vi "Performance Test.vi"() -> ()   [LabVIEW 2021]
uses:
  ChannelCommon/typedef/Benchmark Stats.ctl
  ChannelCommon/typedef/Datatype Waveform.ctl
  CIFChannels/Typedef/Direction.ctl
  ChannelCommon/typedef/FIFO Config.ctl
  CIF_NIChn_FIFO_DAQ_DVR.lvclass
  D:/dev/Packages/Channel_Manager/src/CIFChannels/CIFChannels.lvclass
  <vilib>/Platform/TimedLoop/XDataNode/timing_clust.ctl
  <vilib>/Platform/TimedLoop/XDataNode/nitl_modes.ctl
  <vilib>/Platform/TimedLoop/XDataNode/wakeup.ctl
  ChannelCommon/typedef/TimeStamps.ctl
  CIFChannels/CIFChannels.lvclass/CIFChannels.ctl
  <vilib>/CIF Foundation/CIF Utilities/Statistics/I64/Stats_I64_CIF_U.lvclass/Stats_I64_CIF_U.ctl
  <vilib>/CIF Foundation/CIF Utilities/DataTypes/Flatten U64.vi
  <vilib>/CIF Foundation/CIF Utilities/Statistics/I64/Get Stats.vi
  <vilib>/Platform/TimedLoop/XDataNode/XDataNode.xnode
  <vilib>/Platform/TimedLoop/XDataNode/XDNodeRunTimeDep.lvlib
  CIFChannels/CIFChannels.lvclass
  ChannelCommon/ChannelCommon.lvlib
panel:
  out "Timeout RW Inline":bool
  out "Write (us) 3":T1
  out "Flatten (us) 3":T1
  out "Data Out":T2[](array[typedef])=[{"measurement"=array[200001 elements], "dT"=43.0, "Timestamp"=2, "Read Lock"=FALSE}, {"measurement"=array[200001 elements], "dT"=34.0, "Timestamp"=1, "Read Lock"=FALSE}]
  out "Read (us) 3":T1
  out "Unflatten (us) 3":T1
  out "Flatten (us) TO":T1
  out "Channel R/W (us) TO":T1
  out "Flatten (us)":T1
  out "Channel R/W (us)":T1
  out "avg TO":dbl
  out "max TO":dbl
  out "timed out? 3":bool
  out "timed out?":bool
  out "avg channel":dbl
  out "max channel":dbl
  out "pass":bool
  out "error out":errorcluster
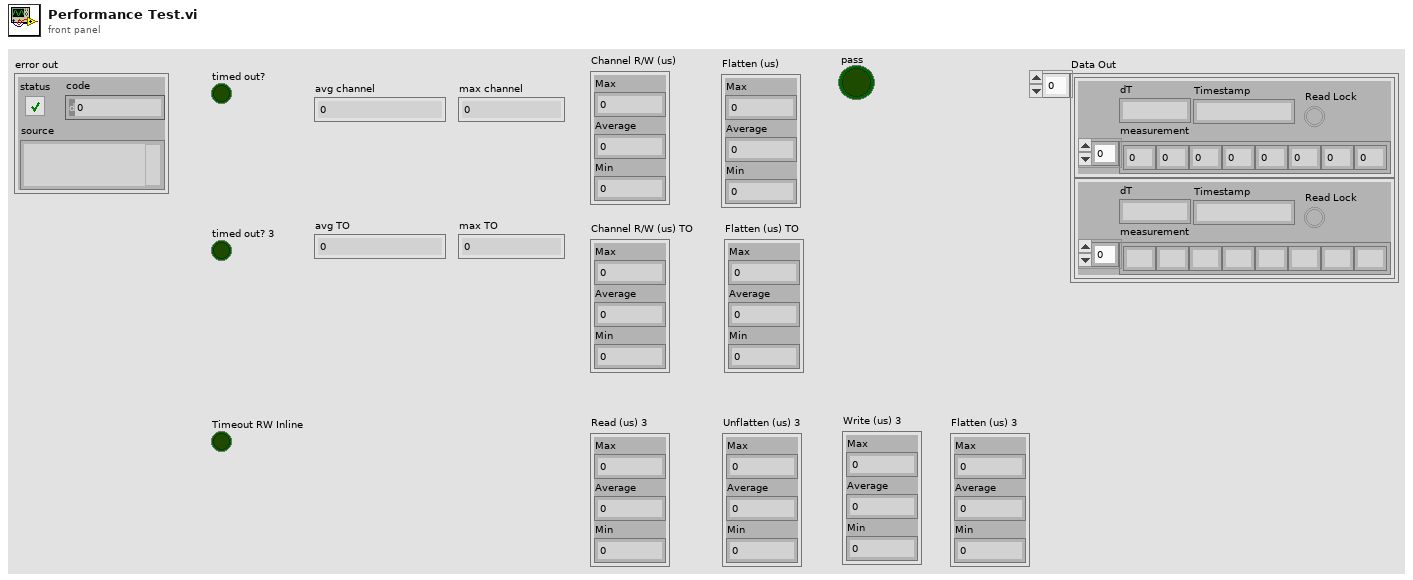
[diagram p1: front panel]
types:
  T1 = typedef "ChannelCommon.lvlib/Benchmark Stats.ctl" = cluster{"Max":i64, "Average":dbl, "Min":i64}
  T2 = typedef "ChannelCommon.lvlib/Datatype Waveform.ctl" = cluster{"measurement":dbl[], "dT":dbl, "Timestamp":i64, "Read Lock":bool}
  T3 = typedef "ChannelCommon.lvlib/FIFO Config.ctl" = cluster{"Max Bytes/Msg":u64, "Max Msg/FIFO":u64, "Flags":u64}
  T4 = typedef "CIFChannels.lvclass/Direction.ctl" = enum16{"Publisher", "Subscriber"}
  T5 = typedef "ChannelCommon.lvlib/TimeStamps.ctl" = cluster{"ClockID":u8, "T0":i64, "T_Out":i64}
  T6 = typedef "XDNodeRunTimeDep.lvlib/timing_clust.ctl" = cluster{"Expected End [f-1]":u64, "Actual End [f-1]":u64, "Finished Late? [f-1]":bool, "Expected End [i-1]":u64, "Actual End [i-1]":u64, "Finished Late? [i-1]":bool, "Expected Start [i]":u64, "Actual Start [i]":u64, "Expected Start [f]":u64, "Actual Start [f]":u64, "Source Name":string, "Structure Name":string, "Period":i64, "Deadline":i64, "Offset":i64, "Start":i64, "Priority":i32, "Timeout":i32, "Mode":T7, "Wakeup Reason":T8, "Error":errorcluster, "Source Type":string, "Secondary Source Type":string, "Global End Time":u64, "Global Start Time":u64, "Frame Duration":u64, "Iteration Duration":u64, "Assigned CPU":i32, "I/O Scan Engine Mode":u32}
  T7 = typedef "XDNodeRunTimeDep.lvlib/nitl_modes.ctl" = enum32{"No Change", "Process missed periods, maintain original phase", "Discard missed periods, maintain original phase", "Process missed periods, ignore original phase", "Discard missed periods, ignore original phase"}
  T8 = typedef "XDNodeRunTimeDep.lvlib/wakeup.ctl" = enum32{"Normal", "Aborted", "Asynchronous wakeup", "Timing source error", "Timed loop error", "Timeout"}
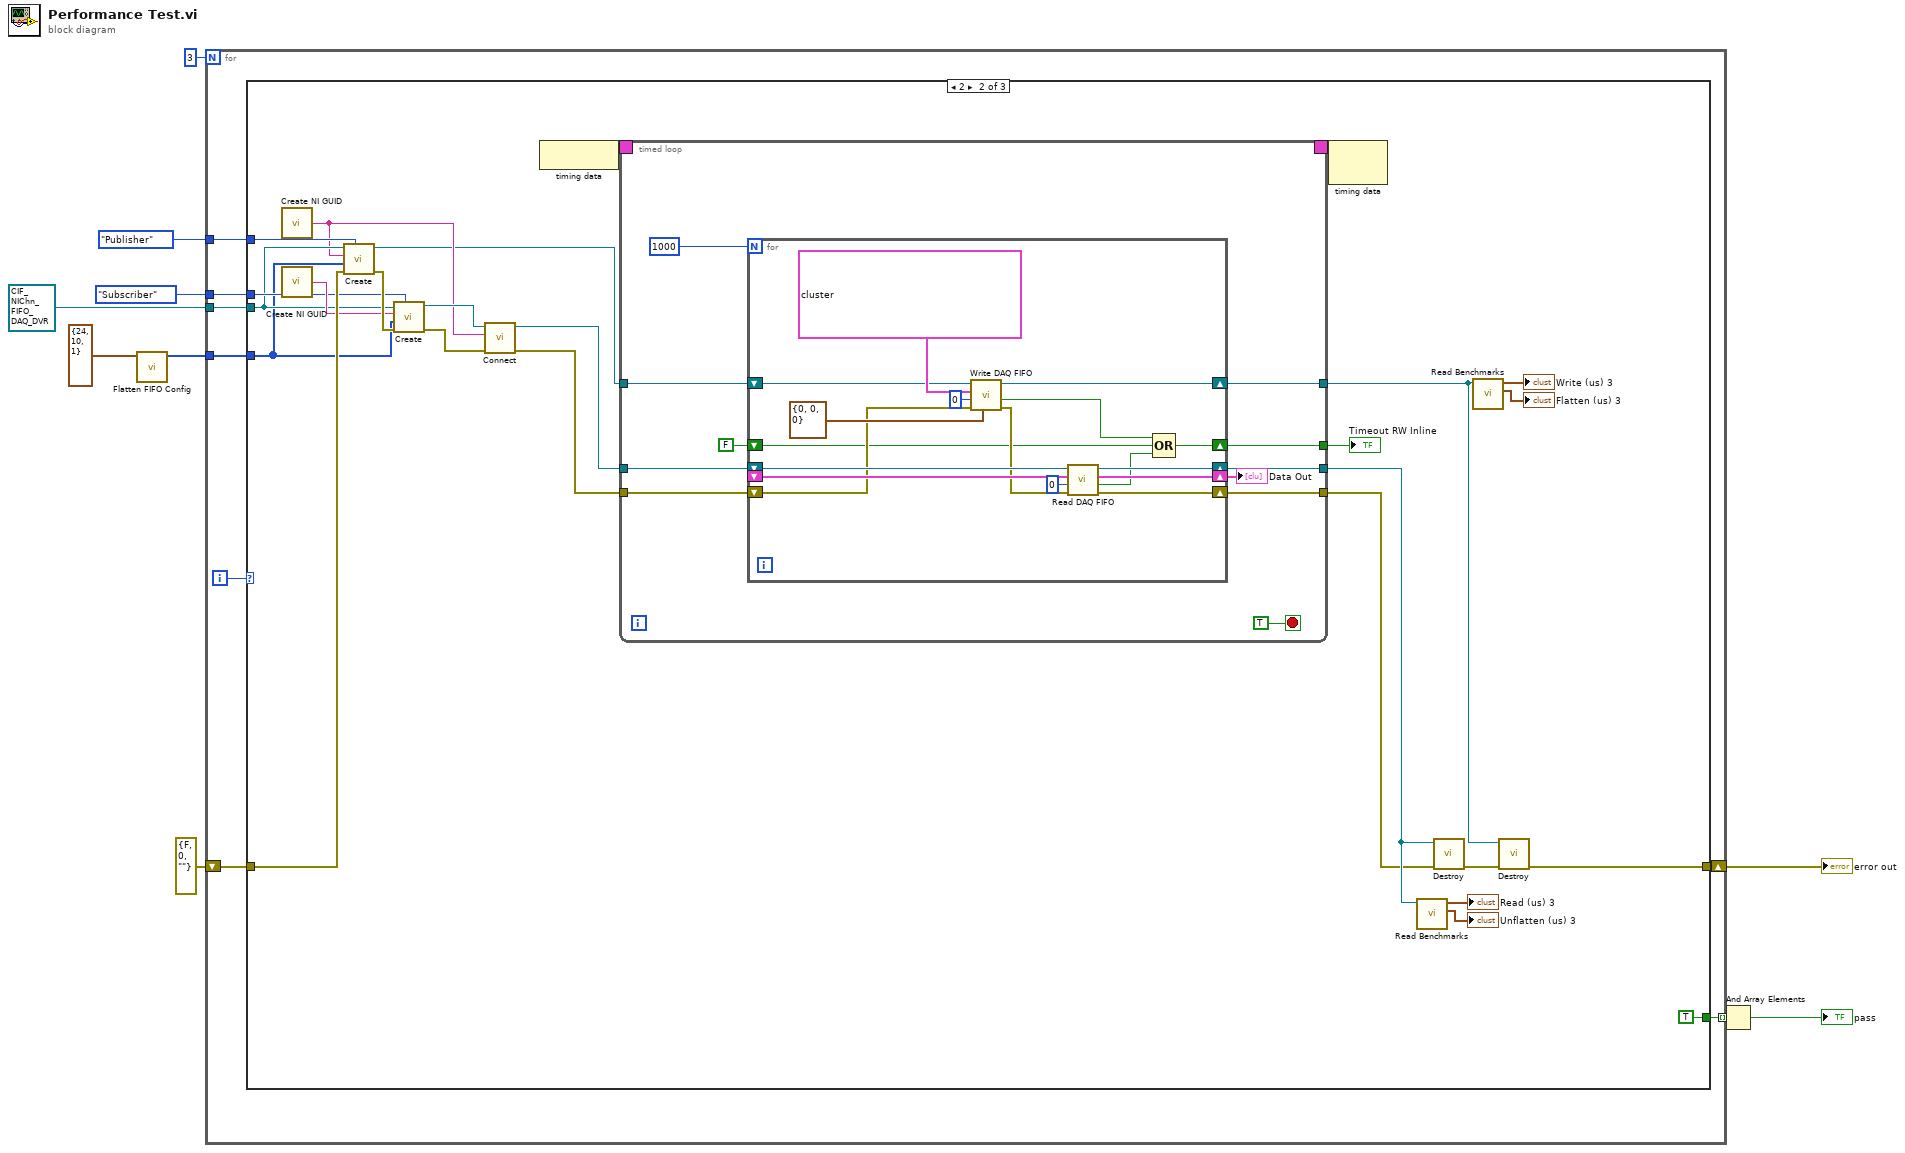
[diagram p0: block diagram]
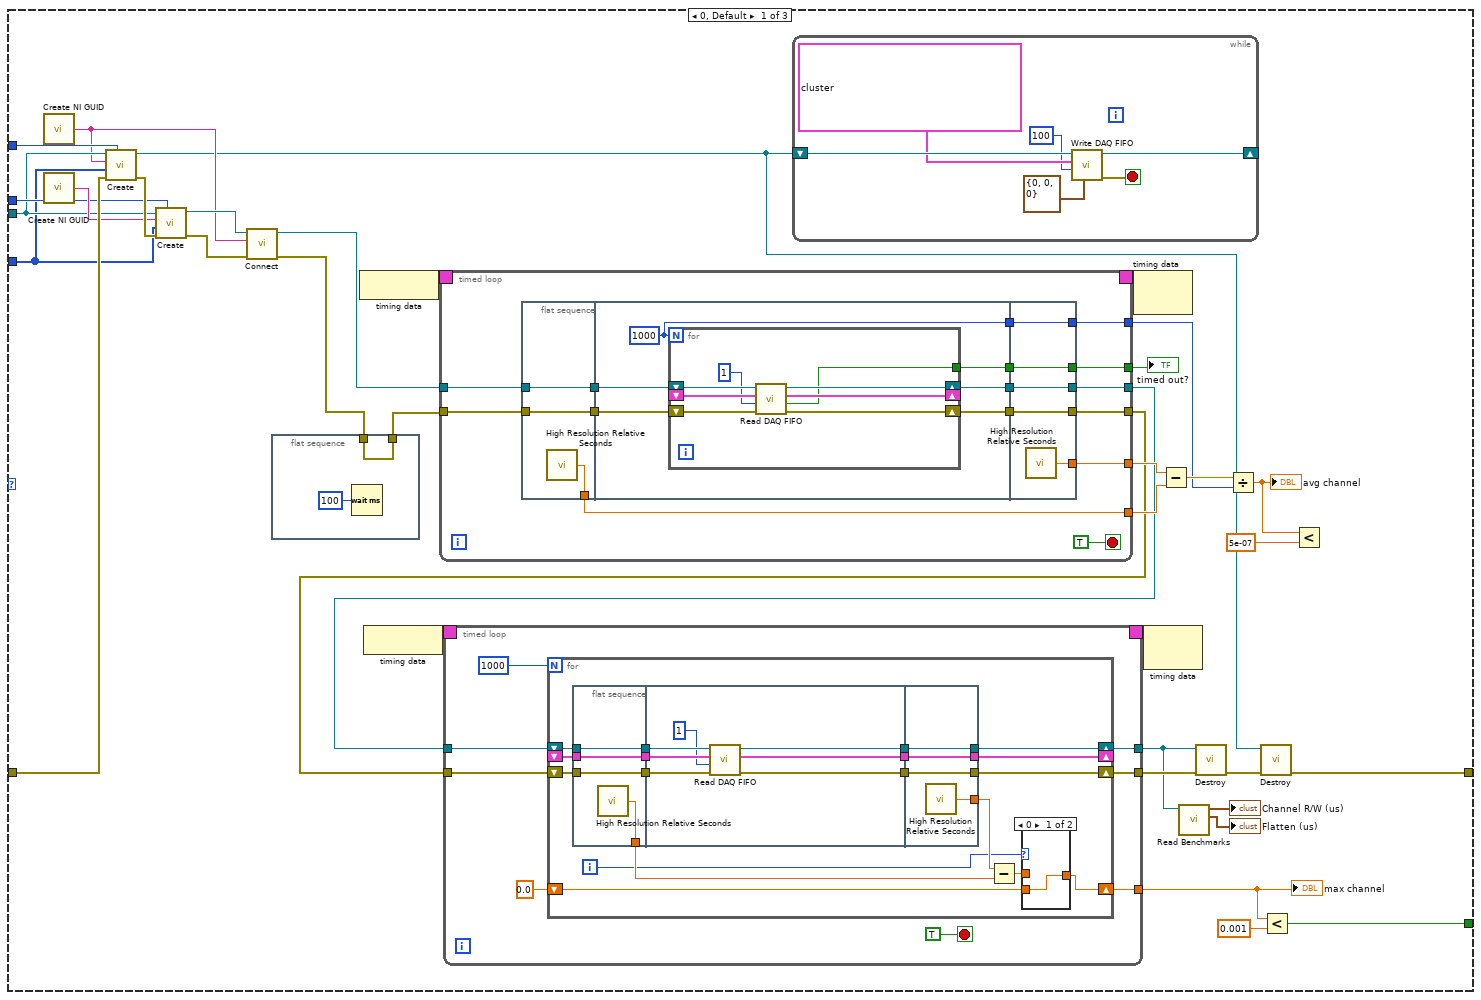
[diagram p2: hidden frame]
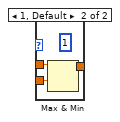
[diagram p3: hidden frame]
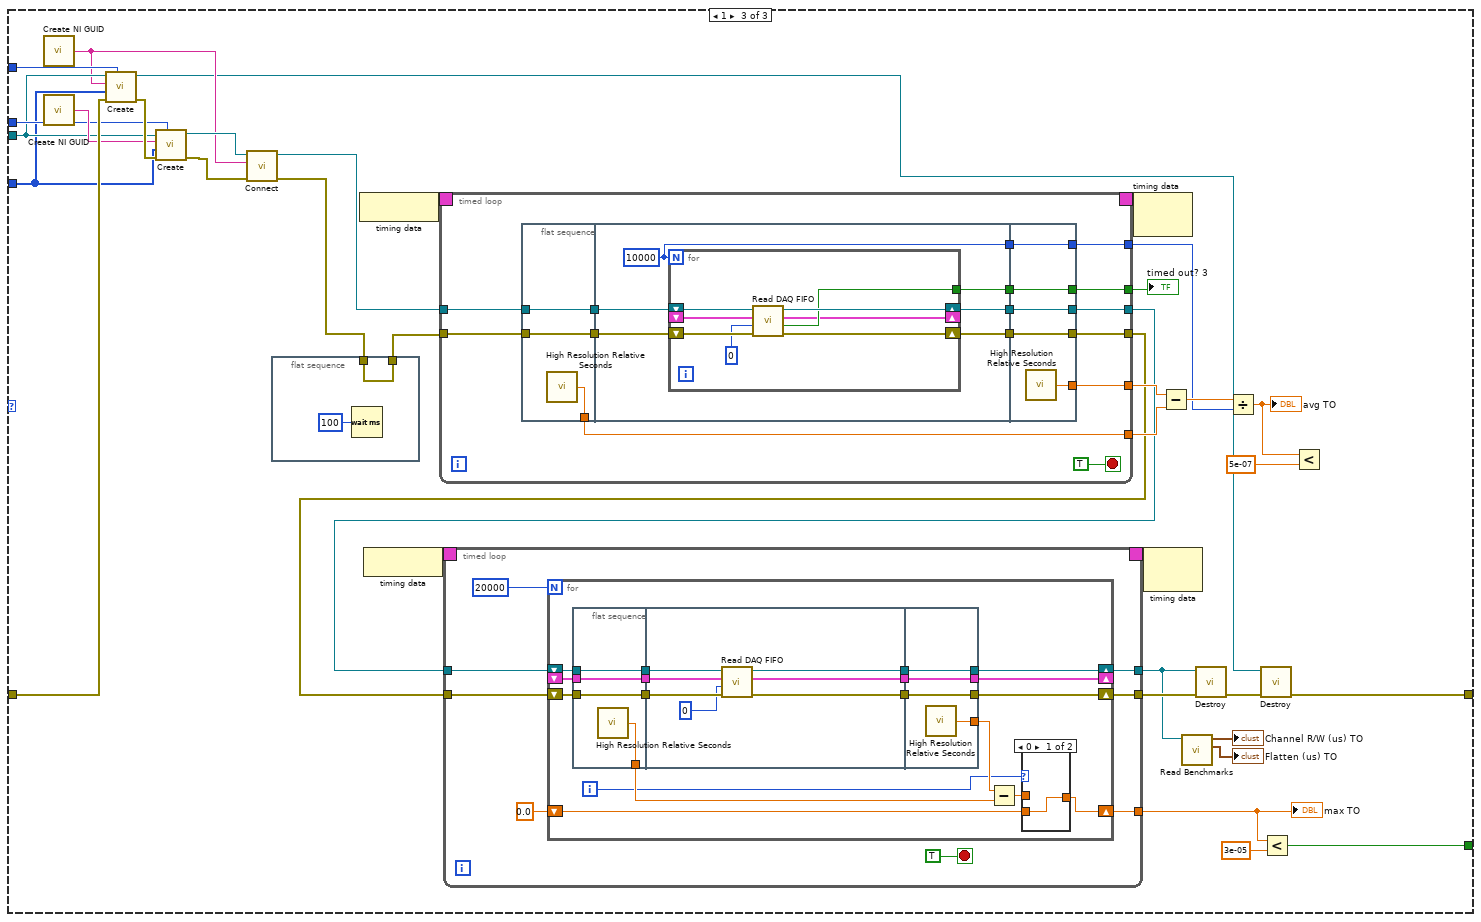
[diagram p4: hidden frame]
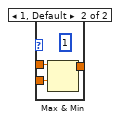
[diagram p5: hidden frame]
diagram:
  n1 = call "Flatten FIFO Config.vi"("FIFO Config in"=T3 {"Max Bytes/Msg"=24, "Max Msg/FIFO"=10, "Flags"=1}) -> ("Flattened FIFO Config"=w2:u8[])  [unwired: 10 in]
  n2 = for {
    N: 3 -> [_]
    tunnel: [w18] -> w8 mode=indexing
    shift-right: [w17] -> w10
    shift-left: errorcluster {"status"=FALSE, "code"=0, "source"=""} ("error out") -> [w15]
    tunnel: Direction."Publisher" ("Direction") -> [w14]
    tunnel: Direction."Subscriber" ("Direction") -> [w13]
    tunnel: refnum<class "CIF_NIChn_FIFO_DAQ_DVR.lvclass"> refnum ("CIF_NIChn_FIFO_DAQ.lvclass") -> [w12]
    tunnel: w2 -> [w11]
    i -> [w16]
    n3 = case shown="2" w16 {
      tunnel: [w40 TRUE w232] -> w18
      tunnel: [w25 w167 w217] -> w17
      tunnel: w15 -> [w38 w177 w230]
      tunnel: w14 -> [w36 w175 w228]
      tunnel: w13 -> [w35 w174 w227]
      tunnel: w12 -> [w34 w173 w226]
      tunnel: w11 -> [w30 w169 w222]
      frame 0, Default {
        n4 = call <vilib>:"Create NI GUID.vi"() -> ("NI GUID"=w32:string)
        n5 = call <vilib>:"Create NI GUID.vi"() -> ("NI GUID"=w37:string)
        n6 = call-dynamic "Create.vi"("Direction"=w36, "error in (no error)"=w38, "Custom Config Data"=w30, "Name"=w32, "CIF_NIChn_FIFO_DAQ in"=w34) -> ("error out"=w39:errorcluster, "CIF_NIChn_FIFO_DAQ out"=w26:refnum<class "CIF_NIChn_FIFO_DAQ_DVR.lvclass">)  [unwired: 5 in]
        n7 = call-dynamic "Create.vi"("Direction"=w35, "error in (no error)"=w39, "Custom Config Data"=w30, "Name"=w37, "CIF_NIChn_FIFO_DAQ in"=w34) -> ("error out"=w31:errorcluster, "CIF_NIChn_FIFO_DAQ out"=w33:refnum<class "CIF_NIChn_FIFO_DAQ_DVR.lvclass">)  [unwired: 5 in]
        n8 = call-dynamic "Connect.vi"("error in (no error)"=w31, "Connection Name"=w32, "CIFTag in"=w33) -> ("error out"=w24:errorcluster, "CIFTag out"=w29:refnum<class "CIF_NIChn_FIFO_DAQ_DVR.lvclass">)  [unwired: 7 in]
        n9 = flat-sequence {
          tunnel: w24 -> [w56]
          tunnel: [w56] -> w23
          frame #0 {
            n10 = Wait (ms)(milliseconds to wait=u32 100) -> ()  [unwired: 1 out]
          }
        }
        n11 = node-c288() -> (w54:T6)
        n12 = node-c288() -> (w52:T6)
        n13 = timed-loop {
          timing: w54 -> [_]
          timing-out: [_] -> w53
          tunnel: w29 -> [w126]
          tunnel: w23 -> [w125]
          tunnel: [w121] -> w46
          tunnel: [w119] -> w45
          tunnel: [w117] -> w50
          tunnel: [w116] -> w49
          tunnel: [w115] -> w47
          tunnel: [w113] -> w22
          stop <- TRUE stop-if-true
          n14 = flat-sequence {
            tunnel: w125 -> [w128]
            tunnel: w126 -> [w129]
            tunnel: [w129] -> w123
            tunnel: [w128] -> w122
            tunnel: [w127] -> w116
            tunnel: w123 -> [w135]
            tunnel: w122 -> [w134]
            tunnel: [w133] -> w120
            tunnel: [w132] -> w118
            tunnel: [w131] -> w114
            tunnel: [w130] -> w112
            tunnel: [w148] -> w121
            tunnel: w120 -> [w148]
            tunnel: [w147] -> w119
            tunnel: w118 -> [w147]
            tunnel: [w146] -> w117
            tunnel: [w145] -> w115
            tunnel: w114 -> [w145]
            tunnel: [w144] -> w113
            tunnel: w112 -> [w144]
            frame #0 {
              n15 = call <vilib>:"High Resolution Relative Seconds.vi"() -> ("relative seconds"=w127:dbl)
            }
            frame #1 {
              w131 = 1000
              n16 = for {
                N: w131 -> [_]
                shift-right: [w138] -> w133
                shift-left: w135 -> [w143]
                shift-right: [w141] -> w132
                shift-left: w134 -> [w142]
                shift-right: [w140] -> _
                shift-left: _ -> [w139]
                tunnel: [w137] -> w130
                n17 = call-dynamic "Read DAQ FIFO.vi"("error in (no error)"=w142, "Timeout (ms)"=1, "Data In"=w139, "CIF_NIChn_FIFO_DAQ in"=w143) -> ("error out"=w141:errorcluster, "timed out?"=w137:bool, "Data Out"=w140:T2[], "CIF_NIChn_FIFO_DAQ out"=w138:refnum<class "CIF_NIChn_FIFO_DAQ_DVR.lvclass">)  [unwired: 3 in, 1 out]
              }
            }
            frame #2 {
              n18 = call <vilib>:"High Resolution Relative Seconds.vi"() -> ("relative seconds"=w146:dbl)
            }
          }
        }
        "timed out?" <- w22
        n19 = timed-loop {
          timing: w52 -> [_]
          timing-out: [_] -> w51
          tunnel: w46 -> [w70]
          tunnel: w45 -> [w69]
          tunnel: [w67] -> w21
          tunnel: [w66] -> w28
          tunnel: [w63] -> w42
          stop <- TRUE stop-if-true
          n20 = for {
            N: 1000 -> [_]
            shift-right: [w82] -> w67
            shift-left: w70 -> [w84]
            shift-right: [w81] -> w66
            shift-left: w69 -> [w83]
            shift-right: [w75] -> w63
            shift-left: 0.0 -> [w76]
            shift-right: [w74] -> _
            shift-left: _ -> [w80]
            i -> [w72]
            n21 = flat-sequence {
              tunnel: w83 -> [w95]
              tunnel: w84 -> [w96]
              tunnel: [w96] -> w88
              tunnel: [w95] -> w87
              tunnel: [w94] -> w78
              tunnel: w80 -> [w93]
              tunnel: [w93] -> w86
              tunnel: w88 -> [w103]
              tunnel: w87 -> [w102]
              tunnel: [w99] -> w85
              tunnel: w86 -> [w98]
              tunnel: [w100] -> w73
              tunnel: [w101] -> w71
              tunnel: [w107] -> w82
              tunnel: w85 -> [w107]
              tunnel: [w106] -> w81
              tunnel: [w105] -> w79
              tunnel: [w104] -> w74
              tunnel: w73 -> [w104]
              tunnel: w71 -> [w106]
              frame #0 {
                n22 = call <vilib>:"High Resolution Relative Seconds.vi"() -> ("relative seconds"=w94:dbl)
              }
              frame #1 {
                n23 = call-dynamic "Read DAQ FIFO.vi"("error in (no error)"=w102, "Timeout (ms)"=1, "Data In"=w98, "CIF_NIChn_FIFO_DAQ in"=w103) -> ("error out"=w101:errorcluster, "Data Out"=w100:T2[], "CIF_NIChn_FIFO_DAQ out"=w99:refnum<class "CIF_NIChn_FIFO_DAQ_DVR.lvclass">)  [unwired: 3 in, 2 out]
              }
              frame #2 {
                n24 = call <vilib>:"High Resolution Relative Seconds.vi"() -> ("relative seconds"=w105:dbl)
              }
            }
            n25 = Subtract(x=w79, y=w78) -> (x-y=w77:dbl)
            n26 = case shown="0" w72 {
              tunnel: w77 -> [_ w92]
              tunnel: w76 -> [w89 w91]
              tunnel: [w89 w90] -> w75
              frame 0 {
              }
              frame 1, Default {
                (unwired) u32 1 ("milliseconds to wait")
                n27 = Max & Min(x=w92, y=w91) -> (max(x,y)=w90:dbl)  [unwired: 1 out]
              }
            }
          }
        }
        "max channel" <- w42
        n28 = while {
          shift-right: [w59] -> _
          shift-left: w26 -> [w62]
          stop <- w60 stop-if-true
          n29 = call-dynamic "Write DAQ FIFO.vi"("FIFO Timestamps"=T5 {"ClockID"=0, "T0"=0, "T_Out"=0}, "Timeout (ms)"=100, "Data In"=T2[] [{"measurement"=array[200001 elements], "dT"=43.0, "Timestamp"=2, "Read Lock"=FALSE}, {"measurement"=array[200001 elements], "dT"=34.0, "Timestamp"=1, "Read Lock"=FALSE}] ("DAQ In"), "CIF_NIChn_FIFO_DAQ in"=w62) -> ("error out"=w60:errorcluster, "CIF_NIChn_FIFO_DAQ out"=w59:refnum<class "CIF_NIChn_FIFO_DAQ_DVR.lvclass">)  [unwired: 4 in, 2 out]
        }
        n30 = node-c288(w53) -> ()  [unwired: 1 out]
        n31 = node-c288(w51) -> ()  [unwired: 1 out]
        n32 = Subtract(x=w50, y=w49) -> (x-y=w48:dbl)
        n33 = call "Read Benchmarks.vi"("CIFChannels in"=w21) -> ("Flatten (us)"=→"Flatten (us)":T1, "Channel R/W (us)"=→"Channel R/W (us)":T1)  [unwired: 9 in]
        n34 = call-dynamic "Destroy.vi"("error in (no error)"=w28, "CIF_NIChn_FIFO_DAQ in"=w21) -> ("error out"=w27:errorcluster)  [unwired: 8 in, 1 out]
        n35 = Divide(x=w48, y=w47) -> (x/y=w44:dbl)
        "avg channel" <- w44
        n36 = call-dynamic "Destroy.vi"("error in (no error)"=w27, "CIF_NIChn_FIFO_DAQ in"=w26) -> ("error out"=w25:errorcluster)  [unwired: 8 in, 1 out]
        n37 = Less?(x=w42, y=0.001) -> (x < y?=w40:bool)
        n38 = Less?(x=w44, y=5e-07) -> ()  [unwired: 1 out]
      }
      frame 2 {
        n39 = call <vilib>:"Create NI GUID.vi"() -> ("NI GUID"=w171:string)
        n40 = call <vilib>:"Create NI GUID.vi"() -> ("NI GUID"=w176:string)
        n41 = call-dynamic "Create.vi"("Direction"=w175, "error in (no error)"=w177, "Custom Config Data"=w169, "Name"=w171, "CIF_NIChn_FIFO_DAQ in"=w173) -> ("error out"=w178:errorcluster, "CIF_NIChn_FIFO_DAQ out"=w162:refnum<class "CIF_NIChn_FIFO_DAQ_DVR.lvclass">)  [unwired: 5 in]
        n42 = call-dynamic "Create.vi"("Direction"=w174, "error in (no error)"=w178, "Custom Config Data"=w169, "Name"=w176, "CIF_NIChn_FIFO_DAQ in"=w173) -> ("error out"=w170:errorcluster, "CIF_NIChn_FIFO_DAQ out"=w172:refnum<class "CIF_NIChn_FIFO_DAQ_DVR.lvclass">)  [unwired: 5 in]
        n43 = call-dynamic "Connect.vi"("error in (no error)"=w170, "Connection Name"=w171, "CIFTag in"=w172) -> ("error out"=w160:errorcluster, "CIFTag out"=w161:refnum<class "CIF_NIChn_FIFO_DAQ_DVR.lvclass">)  [unwired: 7 in]
        n44 = node-c288() -> (w164:T6)
        n45 = timed-loop {
          timing: w164 -> [_]
          timing-out: [_] -> w163
          tunnel: w161 -> [w189]
          tunnel: w160 -> [w188]
          tunnel: [w186] -> w159
          tunnel: [w185] -> w158
          tunnel: [w180] -> w153
          tunnel: w162 -> [w183]
          tunnel: [w182] -> w155
          stop <- TRUE stop-if-true
          n46 = for {
            N: 1000 -> [_]
            shift-right: [w202] -> w186
            shift-left: w189 -> [w206]
            shift-right: [w205] -> w185
            shift-left: w188 -> [w199]
            shift-right: [w204] -> w179
            shift-left: _ -> [w203]
            shift-right: [w196] -> w182
            shift-left: w183 -> [w197]
            shift-right: [w191] -> w180
            shift-left: FALSE -> [w192]
            n47 = call-dynamic "Write DAQ FIFO.vi"("FIFO Timestamps"=T5 {"ClockID"=0, "T0"=0, "T_Out"=0}, "error in (no error)"=w199, "Timeout (ms)"=0, "Data In"=T2[] [{"measurement"=array[200001 elements], "dT"=43.0, "Timestamp"=2, "Read Lock"=FALSE}, {"measurement"=array[200001 elements], "dT"=34.0, "Timestamp"=1, "Read Lock"=FALSE}] ("DAQ In"), "CIF_NIChn_FIFO_DAQ in"=w197) -> ("error out"=w198:errorcluster, "timed out?"=w190:bool, "CIF_NIChn_FIFO_DAQ out"=w196:refnum<class "CIF_NIChn_FIFO_DAQ_DVR.lvclass">)  [unwired: 3 in, 1 out]
            n48 = call-dynamic "Read DAQ FIFO.vi"("error in (no error)"=w198, "Timeout (ms)"=0, "Data In"=w203, "CIF_NIChn_FIFO_DAQ in"=w206) -> ("error out"=w205:errorcluster, "timed out?"=w193:bool, "Data Out"=w204:T2[], "CIF_NIChn_FIFO_DAQ out"=w202:refnum<class "CIF_NIChn_FIFO_DAQ_DVR.lvclass">)  [unwired: 3 in, 1 out]
            n49 = Compound Arithmetic op=OR(w190, w192, w193) -> (w191:bool)
          }
          "Data Out" <- w179
        }
        "Timeout RW Inline" <- w153
        n50 = node-c288(w163) -> ()  [unwired: 1 out]
        n51 = call "Read Benchmarks.vi"("CIFChannels in"=w159) -> ("Flatten (us)"=→"Unflatten (us) 3":T1, "Channel R/W (us)"=→"Read (us) 3":T1)  [unwired: 9 in]
        n52 = call-dynamic "Destroy.vi"("error in (no error)"=w158, "CIF_NIChn_FIFO_DAQ in"=w159) -> ("error out"=w168:errorcluster)  [unwired: 8 in, 1 out]
        n53 = call "Read Benchmarks.vi"("CIFChannels in"=w155) -> ("Flatten (us)"=→"Flatten (us) 3":T1, "Channel R/W (us)"=→"Write (us) 3":T1)  [unwired: 9 in]
        n54 = call-dynamic "Destroy.vi"("error in (no error)"=w168, "CIF_NIChn_FIFO_DAQ in"=w155) -> ("error out"=w167:errorcluster)  [unwired: 8 in, 1 out]
      }
      frame 1 {
        n55 = call <vilib>:"Create NI GUID.vi"() -> ("NI GUID"=w224:string)
        n56 = call <vilib>:"Create NI GUID.vi"() -> ("NI GUID"=w229:string)
        n57 = call-dynamic "Create.vi"("Direction"=w228, "error in (no error)"=w230, "Custom Config Data"=w222, "Name"=w224, "CIF_NIChn_FIFO_DAQ in"=w226) -> ("error out"=w231:errorcluster, "CIF_NIChn_FIFO_DAQ out"=w218:refnum<class "CIF_NIChn_FIFO_DAQ_DVR.lvclass">)  [unwired: 5 in]
        n58 = call-dynamic "Create.vi"("Direction"=w227, "error in (no error)"=w231, "Custom Config Data"=w222, "Name"=w229, "CIF_NIChn_FIFO_DAQ in"=w226) -> ("error out"=w223:errorcluster, "CIF_NIChn_FIFO_DAQ out"=w225:refnum<class "CIF_NIChn_FIFO_DAQ_DVR.lvclass">)  [unwired: 5 in]
        n59 = call-dynamic "Connect.vi"("error in (no error)"=w223, "Connection Name"=w224, "CIFTag in"=w225) -> ("error out"=w216:errorcluster, "CIFTag out"=w221:refnum<class "CIF_NIChn_FIFO_DAQ_DVR.lvclass">)  [unwired: 7 in]
        n60 = flat-sequence {
          tunnel: w216 -> [w248]
          tunnel: [w248] -> w215
          frame #0 {
            n61 = Wait (ms)(milliseconds to wait=u32 100) -> ()  [unwired: 1 out]
          }
        }
        n62 = node-c288() -> (w246:T6)
        n63 = node-c288() -> (w244:T6)
        n64 = timed-loop {
          timing: w246 -> [_]
          timing-out: [_] -> w245
          tunnel: w221 -> [w312]
          tunnel: w215 -> [w311]
          tunnel: [w307] -> w238
          tunnel: [w305] -> w237
          tunnel: [w303] -> w242
          tunnel: [w302] -> w241
          tunnel: [w301] -> w239
          tunnel: [w299] -> w214
          stop <- TRUE stop-if-true
          n65 = flat-sequence {
            tunnel: w311 -> [w314]
            tunnel: w312 -> [w315]
            tunnel: [w315] -> w309
            tunnel: [w314] -> w308
            tunnel: [w313] -> w302
            tunnel: w309 -> [w321]
            tunnel: w308 -> [w320]
            tunnel: [w319] -> w306
            tunnel: [w318] -> w304
            tunnel: [w317] -> w300
            tunnel: [w316] -> w298
            tunnel: [w334] -> w307
            tunnel: w306 -> [w334]
            tunnel: [w333] -> w305
            tunnel: w304 -> [w333]
            tunnel: [w332] -> w303
            tunnel: [w331] -> w301
            tunnel: w300 -> [w331]
            tunnel: [w330] -> w299
            tunnel: w298 -> [w330]
            frame #0 {
              n66 = call <vilib>:"High Resolution Relative Seconds.vi"() -> ("relative seconds"=w313:dbl)
            }
            frame #1 {
              w317 = 10000
              n67 = for {
                N: w317 -> [_]
                shift-right: [w326] -> w319
                shift-left: w321 -> [w329]
                shift-right: [w327] -> w318
                shift-left: w320 -> [w328]
                shift-right: [w324] -> _
                shift-left: _ -> [w323]
                tunnel: [w325] -> w316
                n68 = call-dynamic "Read DAQ FIFO.vi"("error in (no error)"=w328, "Timeout (ms)"=0, "Data In"=w323, "CIF_NIChn_FIFO_DAQ in"=w329) -> ("error out"=w327:errorcluster, "timed out?"=w325:bool, "Data Out"=w324:T2[], "CIF_NIChn_FIFO_DAQ out"=w326:refnum<class "CIF_NIChn_FIFO_DAQ_DVR.lvclass">)  [unwired: 3 in, 1 out]
              }
            }
            frame #2 {
              n69 = call <vilib>:"High Resolution Relative Seconds.vi"() -> ("relative seconds"=w332:dbl)
            }
          }
        }
        "timed out? 3" <- w214
        n70 = timed-loop {
          timing: w244 -> [_]
          timing-out: [_] -> w243
          tunnel: w238 -> [w256]
          tunnel: w237 -> [w255]
          tunnel: [w253] -> w211
          tunnel: [w252] -> w220
          tunnel: [w249] -> w234
          stop <- TRUE stop-if-true
          n71 = for {
            N: 20000 -> [_]
            shift-right: [w268] -> w253
            shift-left: w256 -> [w270]
            shift-right: [w267] -> w252
            shift-left: w255 -> [w269]
            shift-right: [w261] -> w249
            shift-left: 0.0 -> [w262]
            shift-right: [w260] -> _
            shift-left: _ -> [w266]
            i -> [w258]
            n72 = flat-sequence {
              tunnel: w269 -> [w281]
              tunnel: w270 -> [w282]
              tunnel: [w282] -> w274
              tunnel: [w281] -> w273
              tunnel: [w280] -> w264
              tunnel: w266 -> [w279]
              tunnel: [w279] -> w272
              tunnel: w274 -> [w289]
              tunnel: w273 -> [w285]
              tunnel: [w288] -> w271
              tunnel: w272 -> [w286]
              tunnel: [w287] -> w259
              tunnel: [w284] -> w257
              tunnel: [w293] -> w268
              tunnel: w271 -> [w293]
              tunnel: [w292] -> w267
              tunnel: [w291] -> w265
              tunnel: [w290] -> w260
              tunnel: w259 -> [w290]
              tunnel: w257 -> [w292]
              frame #0 {
                n73 = call <vilib>:"High Resolution Relative Seconds.vi"() -> ("relative seconds"=w280:dbl)
              }
              frame #1 {
                n74 = call-dynamic "Read DAQ FIFO.vi"("error in (no error)"=w285, "Timeout (ms)"=0, "Data In"=w286, "CIF_NIChn_FIFO_DAQ in"=w289) -> ("error out"=w284:errorcluster, "Data Out"=w287:T2[], "CIF_NIChn_FIFO_DAQ out"=w288:refnum<class "CIF_NIChn_FIFO_DAQ_DVR.lvclass">)  [unwired: 3 in, 2 out]
              }
              frame #2 {
                n75 = call <vilib>:"High Resolution Relative Seconds.vi"() -> ("relative seconds"=w291:dbl)
              }
            }
            n76 = Subtract(x=w265, y=w264) -> (x-y=w263:dbl)
            n77 = case shown="0" w258 {
              tunnel: w263 -> [_ w278]
              tunnel: w262 -> [w275 w277]
              tunnel: [w275 w276] -> w261
              frame 0 {
              }
              frame 1, Default {
                (unwired) u32 1 ("milliseconds to wait")
                n78 = Max & Min(x=w278, y=w277) -> (max(x,y)=w276:dbl)  [unwired: 1 out]
              }
            }
          }
        }
        "max TO" <- w234
        n79 = node-c288(w245) -> ()  [unwired: 1 out]
        n80 = node-c288(w243) -> ()  [unwired: 1 out]
        n81 = Subtract(x=w242, y=w241) -> (x-y=w240:dbl)
        n82 = call "Read Benchmarks.vi"("CIFChannels in"=w211) -> ("Flatten (us)"=→"Flatten (us) TO":T1, "Channel R/W (us)"=→"Channel R/W (us) TO":T1)  [unwired: 9 in]
        n83 = call-dynamic "Destroy.vi"("error in (no error)"=w220, "CIF_NIChn_FIFO_DAQ in"=w211) -> ("error out"=w219:errorcluster)  [unwired: 8 in, 1 out]
        n84 = Divide(x=w240, y=w239) -> (x/y=w236:dbl)
        "avg TO" <- w236
        n85 = call-dynamic "Destroy.vi"("error in (no error)"=w219, "CIF_NIChn_FIFO_DAQ in"=w218) -> ("error out"=w217:errorcluster)  [unwired: 8 in, 1 out]
        n86 = Less?(x=w234, y=3e-05) -> (x < y?=w232:bool)
        n87 = Less?(x=w236, y=5e-07) -> ()  [unwired: 1 out]
      }
    }
  }
  "error out" <- w10
  n88 = And Array Elements(Boolean array=w8) -> (logical AND=→"pass":bool)
